vi "GetGXMLCfgStrain.vi"(8 "error in (no error)":errorcluster, 11 "Strain in":refnum<class "Strain.lvclass">) -> (0 "error out":errorcluster, 2 "StrainChanCfg":T1, 3 "Strain out":refnum<class "Strain.lvclass">)   [LabVIEW 2012, in "Measurement Channels.lvlib" / "Strain.lvclass"]
uses:
  Strain.lvclass
  StrainProps_TD.ctl
  Strain.lvclass/Strain.ctl
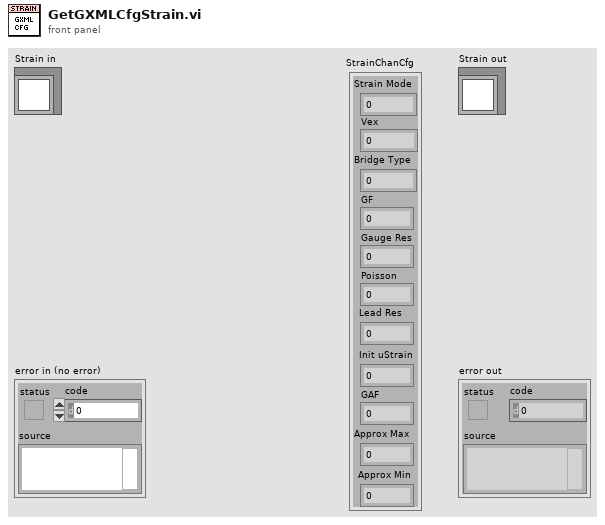
[diagram p1: front panel]
types:
  T1 = typedef "Measurement Channels.lvlib/Strain.lvclass/StrainProps_TD.ctl" = cluster{"Strain Mode":u16, "Vex":dbl, "Bridge Type":u16, "GF":dbl, "Gauge Res":i32, "Poisson":dbl, "Lead Res":dbl, "Init uStrain":dbl, "GAF":dbl, "Approx Max":dbl, "Approx Min":dbl}
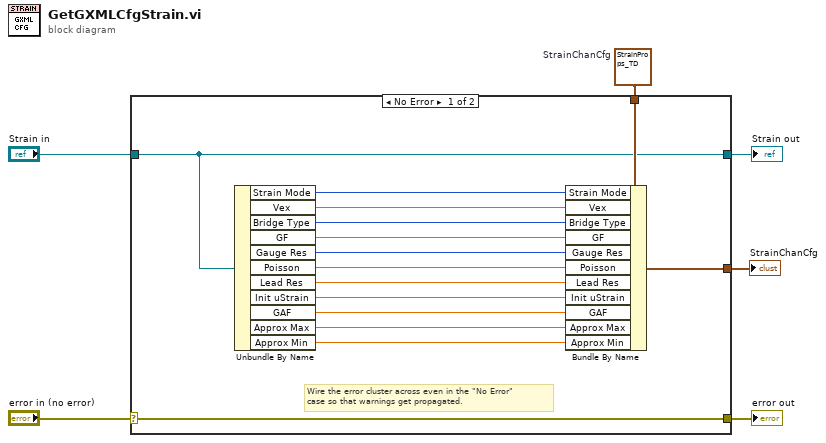
[diagram p0: block diagram]
diagram:
  w2 = T1 {"Strain Mode"=0, "Vex"=0.0, "Bridge Type"=0, "GF"=0.0, "Gauge Res"=0, "Poisson"=0.0, "Lead Res"=0.0, "Init uStrain"=0.0, "GAF"=0.0, "Approx Max"=0.0, "Approx Min"=0.0}  # StrainChanCfg
  n1 = case shown="No Error" "error in (no error)" {
    selector: "error in (no error)" -> [w21 w24]
    tunnel: [w21 w24] -> w5
    tunnel: [w19 w23] -> w3
    tunnel: "Strain in" -> [w19 w23]
    tunnel: w2 -> [w20 w22]
    tunnel: [w7 w22] -> w1
    frame No Error {
      # "Wire the error cluster across even in the \"No Error\"\ncase so that warnings get propagated."
      n2 = Unbundle By Name(w19) -> ("Strain Mode"=w18:u16, "Vex"=w17:dbl, "Bridge Type"=w16:u16, "GF"=w15:dbl, "Gauge Res"=w14:i32, "Poisson"=w13:dbl, "Lead Res"=w12:dbl, "Init uStrain"=w11:dbl, "GAF"=w10:dbl, "Approx Max"=w9:dbl, "Approx Min"=w8:dbl)
      n3 = Bundle By Name(cluster=w20, "Strain Mode"=w18, "Vex"=w17, "Bridge Type"=w16, "GF"=w15, "Gauge Res"=w14, "Poisson"=w13, "Lead Res"=w12, "Init uStrain"=w11, "GAF"=w10, "Approx Max"=w9, "Approx Min"=w8) -> (w7:T1)
    }
    frame Error {
    }
  }
  "error out" <- w5
  "Strain out" <- w3
  "StrainChanCfg" <- w1
